vi "01b-add_two_numbers.vi"() -> ()   [LabVIEW 2018, in "LV2Julia_examples.lvlib"]
uses:
  LV2Julia_examples.lvlib
  LV2Julia_core/VIs/Server or client state.ctl
  LV2Julia_core/VIs/detailed error info.ctl
  LV2Julia_core/VIs/StackFrame.ctl
  LV2Julia_core/VIs/Commands.ctl
  f710999a-539f-4856-b26e-0dc164bcc35a.vi
  f710999a-539f-4856-b26e-0dc164bcc35a.vi/d79e82fc-0f39-47ea-8721-7ab07cf6f2de.vi
  f710999a-539f-4856-b26e-0dc164bcc35a.vi/d79e82fc-0f39-47ea-8721-7ab07cf6f2de.vi/9dc38c00-9d3d-4b5a-b423-a9ea6f4850be.vi
  f710999a-539f-4856-b26e-0dc164bcc35a.vi/d79e82fc-0f39-47ea-8721-7ab07cf6f2de.vi/c9a7705c-deb9-4de6-a30a-59d3cc1926e2.vi
  f710999a-539f-4856-b26e-0dc164bcc35a.vi/d79e82fc-0f39-47ea-8721-7ab07cf6f2de.vi/0cf201d5-1e3b-47af-ba65-f2904eccdfec.vi
  LV2Julia_core/VIs/jl-scripts path.vi
  LV2Julia_core/VIs/check ID validity.vi
  LV2Julia_core/VIs/bindata_descr to JSON.vi
  LV2Julia_core/VIs/check cluster field names.vi
  LV2Julia_core/VIs/concat JSON.vi
  LV2Julia_core/VIs/build request.vi
  LV2Julia_core/VIs/Parse server response.vi
  LV2Julia_core/VIs/log jl exceptions.vi
  LV2Julia_core/LV2Julia_core.lvlib
panel:
  in  "y":dbl=2.0
  in  "x":dbl=2.0
  in  "next":bool
  out "x+y":dbl=nan
  out "detailed error info":T1
  out "current error":errorcluster
  out "final error":errorcluster
  out "short err code":u8
  in  "stop":bool
  out "ZMQ timeout":bool
  out "Julia script file path":path
  out "temporary script path":path
  out "Jl Server state":T3
  # "This VI is slightly different from the previous example (see the wiring diagramm), but uses the same julia script."
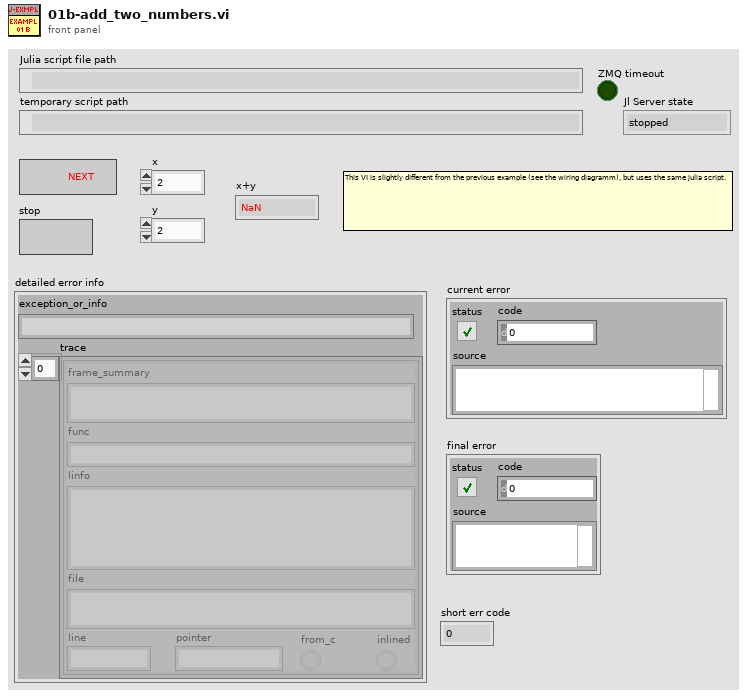
[diagram p1: front panel]
types:
  T1 = typedef "LV2Julia_core.lvlib/detailed error info.ctl" = cluster{"exception_or_info":string, "trace":T2[]}
  T2 = typedef "LV2Julia_core.lvlib/StackFrame.ctl" = cluster{"frame_summary":string, "func":string, "linfo":string, "file":string, "line":i32, "pointer":u64, "from_c":bool, "inlined":bool}
  T3 = typedef "LV2Julia_core.lvlib/Server or client state.ctl" = enum16{"stopped", "running", "unknown"}
  T4 = typedef "LV2Julia_core.lvlib/Commands.ctl" = enum16{"Start Jl-server & Init LV-client", "Send request & Get response ", "Stop Jl-server & Cleanup LV-client", "Cleanup LV-client", "Start Jl-server", "Stop Jl-server", "Init LV-Client", "Cleanup LV-Client", "(not allowed)", "Set LV Client state", "Set Jl Server state", "set ZMQ timeout", "read ZMQ timeout", "read-out state"}
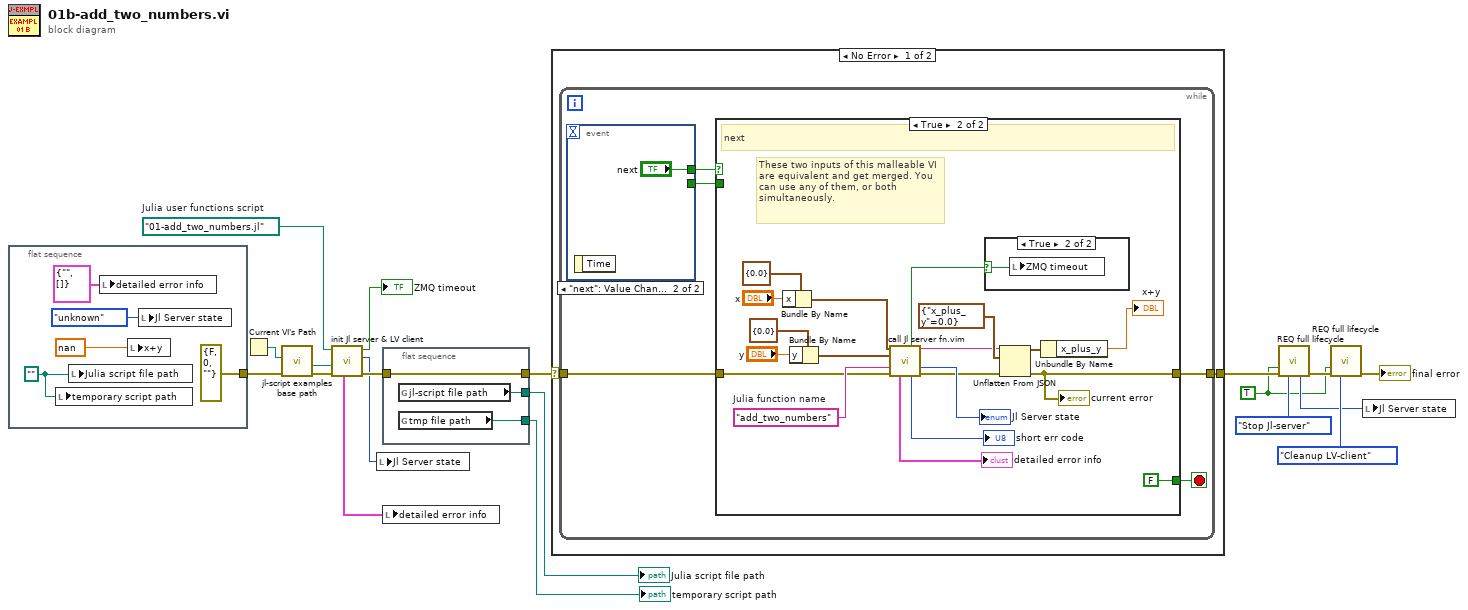
[diagram p0: block diagram]
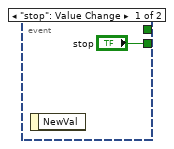
[diagram p2: hidden frame]
diagram:
  w9 = path "01-add_two_numbers.jl"  # Julia user functions script
  w10 = TRUE ("Force command")
  n1 = flat-sequence {
    tunnel: [errorcluster {"status"=FALSE, "code"=0, "source"=""} ("error in (no error)")] -> w4
    frame #0 {
      w20 = path ""
      n2 = local write "temporary script path"(w20) -> ()
      n3 = local write "Julia script file path"(w20) -> ()
      n4 = local write "detailed error info"(T1 {"exception_or_info"="", "trace"=[]} ("detailed error info")) -> ()
      n5 = local write "x+y"(nan ("Server response")) -> ()
      n6 = local write "Jl Server state"(Server_or_client_state."unknown" ("Jl Server state out")) -> ()
    }
  }
  n7 = Current VI's Path() -> (path=w5:path)
  n8 = call "jl-script examples base path.vi"("error in (no error)"=w4, "calling example VI path"=w5) -> ("error out"=w3:errorcluster, "jl-script-examples base path"=w2:path)  [unwired: 8 in]
  n9 = call "init Jl server & LV client.vi"("error in (no error)"=w3, "Base path (not a path)"=w2, "Julia user functions script"=w9) -> ("error out"=w8:errorcluster, "Jl Server state out"=w6:T3, "timeout?"=→"ZMQ timeout":bool, "detailed error info"=w1:T1)  [unwired: 3 in, 2 out]
  n10 = local write "Jl Server state"(w6) -> ()
  n11 = flat-sequence {
    tunnel: [w27] -> w14
    tunnel: w8 -> [w27]
    tunnel: [w26] -> w12
    tunnel: [w25] -> w13
    frame #0 {
      n12 = global read "jl-scripts path.vi" "jl-script file path"() -> (w26:path)
      n13 = global read "jl-scripts path.vi" "tmp file path"() -> (w25:path)
    }
  }
  n14 = local write "detailed error info"(w1) -> ()
  n15 = case shown="No Error" w14 {
    selector: w14 -> [w28 w59]
    tunnel: [w29 w59] -> w19
    frame No Error {
      n16 = while {
        tunnel: w28 -> [w33]
        tunnel: [w34] -> w29
        stop <- w31 stop-if-true
        n17 = event shown="[1] \"next\": Value Change" {
          selector: _ -> [_ _]
          dyn-events: _ -> [_ _]
          timeout: _ -> [_ _]
          tunnel: [_ "next"] -> w32
          tunnel: ["stop" _] -> w30
          event "stop": Value Change {
            n18 = event-data() -> ()  [unwired: 1 in, 1 out]
          }
          event "next": Value Change {
            n19 = event-data() -> ()  [unwired: 1 in, 1 out]
          }
        }
        n20 = case shown="True" w32 {
          tunnel: [w38 w54] -> w34
          tunnel: w33 -> [w38 w46]
          tunnel: [w37 FALSE ("stop this VI only")] -> w31
          tunnel: w30 -> [w37 _]
          frame False {
            # "stop"
          }
          frame True {
            w47 = "add_two_numbers"  # Julia function name
            # "These two inputs of this malleable VI are equivalent and get merged. You can use any of them, or both simultaneously."
            # "next"
            n21 = Bundle By Name(cluster=cluster{"x":dbl} {"x"=0.0}, "x"="x") -> (w41:cluster{"x":dbl})
            n22 = Bundle By Name(cluster=cluster{"y":dbl} {"y"=0.0}, "y"="y") -> (w42:cluster{"y":dbl})
            n23 = call "call Jl server fn.vim"("Arguments 1"=w41, "Arguments 2"=w42, "fun2call"=w47, "error in (no error)"=w46) -> ("timeout?"=w44:bool, "JSON received"=w39:string, "Jl Server state out"=→"Jl Server state":T3, "detailed error info"=→"detailed error info":T1, "return code"=→"short err code":u8, "error out"=w40:errorcluster)  [unwired: 5 in, 1 out]
            n24 = case shown="True" w44 {
              selector: w44 -> [_ w58]
              frame False {
              }
              frame True {
                n25 = local write "ZMQ timeout"(w58) -> ()
              }
            }
            n26 = Unflatten From JSON(JSON string=w39, type and defaults=cluster{"x_plus_y":dbl} {"x_plus_y"=0.0} ("parsed response"), error in (no error)=w40) -> (value=w56:cluster{"x_plus_y":dbl}, error out=w54:errorcluster)  [unwired: 4 in]
            "current error" <- w54
            n27 = Unbundle By Name(w56) -> ("x_plus_y"=→"x+y":dbl)
          }
        }
      }
    }
    frame Error {
    }
  }
  n28 = call "REQ full lifecycle.vi"("Force command"=w10, "error in"=w19, "command"=Commands."Stop Jl-server") -> ("Jl Server state out"=w11:T3, "error out"=w17:errorcluster)  [unwired: 6 in, 5 out]
  n29 = call "REQ full lifecycle.vi"("Force command"=w10, "error in"=w17, "command"=Commands."Cleanup LV-client") -> ("error out"=→"final error":errorcluster)  [unwired: 6 in, 6 out]
  n30 = local write "Jl Server state"(w11) -> ()
  "temporary script path" <- w13
  "Julia script file path" <- w12
